vi "Camera Test Suite.vi"() -> ()   [LabVIEW 2015]
panel:
  out "Status":T1
  in  "Exposure":dbl=0.1
  in  "Save location":path
  out "Image":T2(plugin-control)
  in  "Test":bool
  in  "stop":bool
  in  "Function to test":T3(ring)
  in  "Camera vi path":path
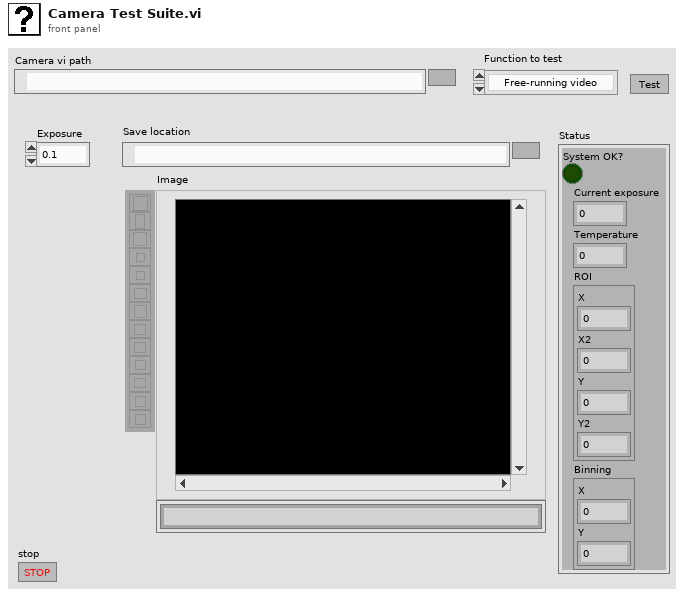
[diagram p1: front panel]
types:
  T1 = cluster{"System OK?":bool, "Current exposure":dbl, "Temperature":dbl, "ROI":cluster{"X":u32, "X2":u32, "Y":u32, "Y2":u32}, "Binning":cluster{"X":u32, "Y":u32}}
  T2 = typedef "IMAQ Image.ctl" = refnum<image>
  T3 = enum16{"Free-running video", "Capture 1 frame", "Capture 10 frames", "Settings", "Change exposure", "Get status"}
  T4 = typedef "Image Type" = u32
  T5 = enum16{"Initialize", "Shut down", "Set capture mode", "Set exposure", "Trigger and read", "Get status", "Other settings"}
  T6 = cluster{"New Image":T2, "Image":refnum<vi>, "FPS target":dbl}
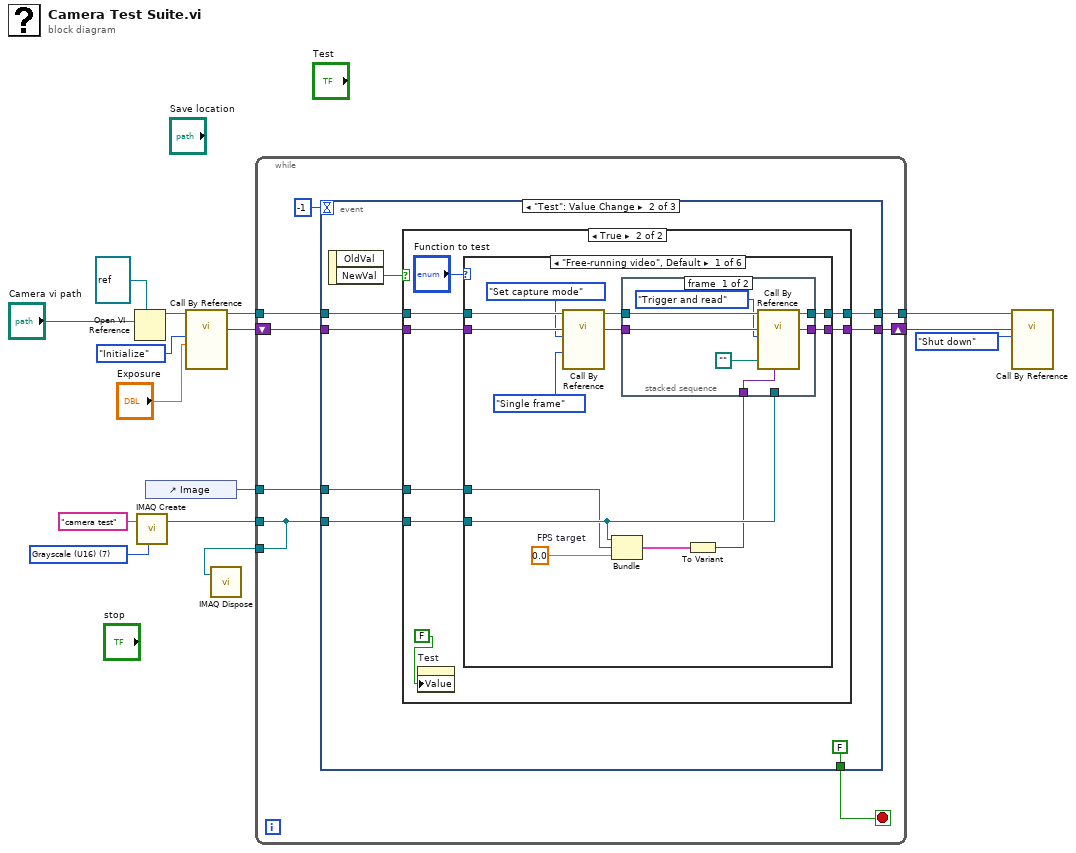
[diagram p0: block diagram]
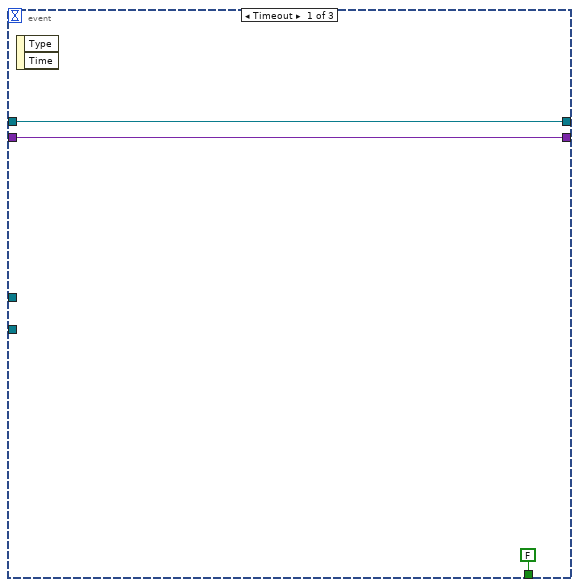
[diagram p2: hidden frame]
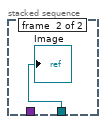
[diagram p4: hidden frame]
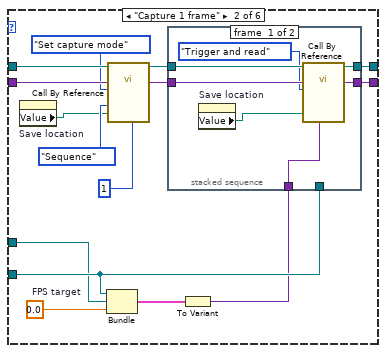
[diagram p5: hidden frame]
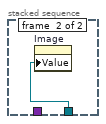
[diagram p6: hidden frame]
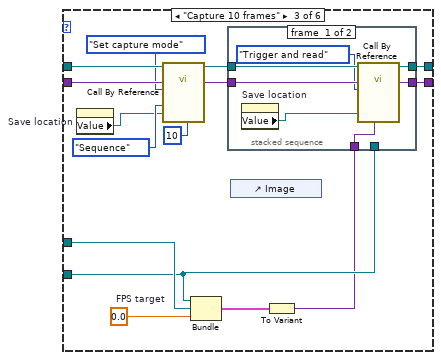
[diagram p7: hidden frame]
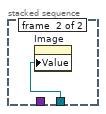
[diagram p8: hidden frame]
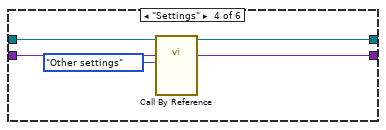
[diagram p9: hidden frame]
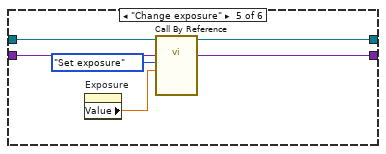
[diagram p10: hidden frame]
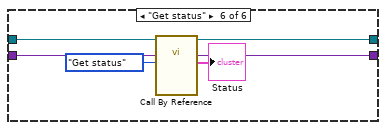
[diagram p11: hidden frame]
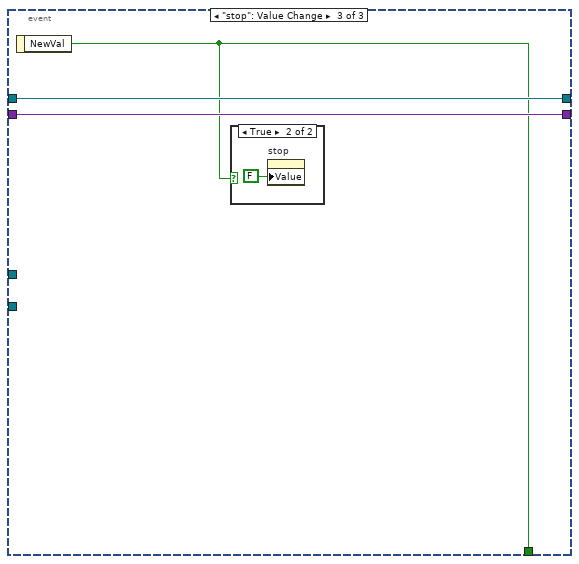
[diagram p12: hidden frame]
diagram:
  w5 = T4 7 items=["Grayscale (U8)", "Grayscale (I16)", "Grayscale (SGL)", "Complex (CSG)", "RGB (U32)", "HSL (U32)", "RGB (U64)", "Grayscale (U16)"] ("Image Type")
  n1 = Open VI Reference(type specifier VI Refnum (for type only)=refnum<vi> refnum, vi path="Camera vi path") -> (vi reference=w13:refnum<vi>)  [unwired: 4 in, 1 out]
  n2 = call "IMAQ Create"("Image Name"="camera test", "Image Type"=w5) -> ("New Image"=w4:T2)  [unwired: 3 in, 1 out]
  n3 = control-ref of="Image"() -> (w1:refnum<vi>)
  n4 = call-by-ref "?"(reference=w13, "Exposure time (s)"="Exposure", "Operation"=T5."Initialize") -> (reference out=w10:refnum<vi>, "Camera-specific out"=w8:variant)  [unwired: 9 in, 2 out]
  n5 = while {
    tunnel: w10 -> [w21]
    tunnel: [w22] -> w12
    shift-right: [w20] -> w7
    shift-left: w8 -> [w19]
    tunnel: w4 -> [w18]
    tunnel: [w18] -> w3
    tunnel: w1 -> [w16]
    stop <- w17 stop-if-true
    n6 = event shown="[1] \"Test\": Value Change" {
      selector: _ -> [_ _ _]
      dyn-events: _ -> [_ _ _]
      timeout: -1 -> [_ _ _]
      tunnel: [w26 w34 w131] -> w22
      tunnel: w21 -> [w26 w33 w131]
      tunnel: [w25 w32 w130] -> w20
      tunnel: w19 -> [w25 w31 w130]
      tunnel: w18 -> [_ w29 _]
      tunnel: [FALSE ("NewVal") FALSE ("NewVal") w129] -> w17
      tunnel: w16 -> [_ w27 _]
      event Timeout {
        n7 = event-data() -> ()  [unwired: 1 in, 2 out]
      }
      event "Test": Value Change {
        n8 = event-data() -> ("NewVal"=w30:bool)  [unwired: 1 in, 1 out]
        n9 = case shown="True" w30 {
          tunnel: [w36 w43] -> w34
          tunnel: w33 -> [w36 w42]
          tunnel: [w35 w41] -> w32
          tunnel: w31 -> [w35 w40]
          tunnel: w29 -> [_ w38]
          tunnel: w27 -> [_ w37]
          frame False {
          }
          frame True {
            n10 = property on="Test" class="Bool (strict)"("Value"=FALSE) -> ()  [unwired: 2 in, 2 out]
            n11 = case shown="\"Free-running video\", Default" "Function to test" {
              tunnel: [w52 w75 w98 w115 w121 w127] -> w43
              tunnel: w42 -> [w57 w80 w103 w116 w122 w128]
              tunnel: [w50 w73 w96 w113 w119 w125] -> w41
              tunnel: w40 -> [w56 w79 w102 w114 w120 w126]
              tunnel: w38 -> [w47 w70 w90 _ _ _]
              tunnel: w37 -> [w46 w69 w91 _ _ _]
              frame "Free-running video", Default {
                w49 = 0.0  # FPS target
                n12 = call-by-ref "?"(reference=w57, "Camera-specific in"=w56, "Capture mode"=enum16{"Single frame", "Sequence"}."Single frame", "Operation"=T5."Set capture mode") -> (reference out=w53:refnum<vi>, "Camera-specific out"=w51:variant)  [unwired: 8 in, 2 out]
                n13 = Bundle("New Image"=w47, "Image"=w46, "FPS target"=w49) -> (w48:T6)  [unwired: 1 in]
                n14 = To Variant(anything=w48) -> (Variant=w45:variant)
                n15 = stacked-sequence {
                  tunnel: w53 -> [w64 _]
                  tunnel: [w63 _] -> w52
                  tunnel: w51 -> [w62 _]
                  tunnel: [w61 _] -> w50
                  tunnel: w47 -> [_ w65]
                  tunnel: w45 -> [w58 _]
                  frame #0 {
                    n16 = call-by-ref "?"(reference=w64, "Image in"=w58, "Camera-specific in"=w62, "Save path"=path "", "Operation"=T5."Trigger and read") -> (reference out=w63:refnum<vi>, "Camera-specific out"=w61:variant)  [unwired: 7 in, 2 out]
                  }
                  frame #1 {
                    "Image" <- w65
                  }
                }
              }
              frame "Capture 1 frame" {
                w68 = 0.0  # FPS target
                n17 = property on="Save location" class="Path"() -> ("Value"=w71:path)  [unwired: 2 in, 2 out]
                n18 = Bundle("New Image"=w70, "Image"=w69, "FPS target"=w68) -> (w67:T6)  [unwired: 1 in]
                n19 = call-by-ref "?"(reference=w80, "Frames in sequence"=u32 1, "Camera-specific in"=w79, "Save path"=w71, "Capture mode"=enum16{"Single frame", "Sequence"}."Sequence", "Operation"=T5."Set capture mode") -> (reference out=w76:refnum<vi>, "Camera-specific out"=w74:variant)  [unwired: 6 in, 2 out]
                n20 = To Variant(anything=w67) -> (Variant=w66:variant)
                n21 = stacked-sequence {
                  tunnel: w76 -> [w87 _]
                  tunnel: [w86 _] -> w75
                  tunnel: w74 -> [w85 _]
                  tunnel: [w84 _] -> w73
                  tunnel: w70 -> [_ w88]
                  tunnel: w66 -> [w81 _]
                  frame #0 {
                    n22 = property on="Save location" class="Path"() -> ("Value"=w82:path)  [unwired: 2 in, 2 out]
                    n23 = call-by-ref "?"(reference=w87, "Image in"=w81, "Camera-specific in"=w85, "Save path"=w82, "Operation"=T5."Trigger and read") -> (reference out=w86:refnum<vi>, "Camera-specific out"=w84:variant)  [unwired: 7 in, 2 out]
                  }
                  frame #1 {
                    n24 = property on="Image" class="ImageControl"("Value"=w88) -> ()  [unwired: 2 in, 2 out]
                  }
                }
              }
              frame "Capture 10 frames" {
                w93 = 0.0  # FPS target
                n25 = property on="Save location" class="Path"() -> ("Value"=w94:path)  [unwired: 2 in, 2 out]
                n26 = call-by-ref "?"(reference=w103, "Frames in sequence"=u32 10, "Camera-specific in"=w102, "Save path"=w94, "Capture mode"=enum16{"Single frame", "Sequence"}."Sequence", "Operation"=T5."Set capture mode") -> (reference out=w99:refnum<vi>, "Camera-specific out"=w97:variant)  [unwired: 6 in, 2 out]
                n27 = Bundle("New Image"=w90, "Image"=w91, "FPS target"=w93) -> (w92:T6)  [unwired: 1 in]
                n28 = control-ref of="Image"() -> ()  [unwired: 1 out]
                n29 = To Variant(anything=w92) -> (Variant=w89:variant)
                n30 = stacked-sequence {
                  tunnel: w99 -> [w110 _]
                  tunnel: [w109 _] -> w98
                  tunnel: w97 -> [w108 _]
                  tunnel: [w107 _] -> w96
                  tunnel: w90 -> [_ w111]
                  tunnel: w89 -> [w104 _]
                  frame #0 {
                    n31 = property on="Save location" class="Path"() -> ("Value"=w105:path)  [unwired: 2 in, 2 out]
                    n32 = call-by-ref "?"(reference=w110, "Image in"=w104, "Camera-specific in"=w108, "Save path"=w105, "Operation"=T5."Trigger and read") -> (reference out=w109:refnum<vi>, "Camera-specific out"=w107:variant)  [unwired: 7 in, 2 out]
                  }
                  frame #1 {
                    n33 = property on="Image" class="ImageControl"("Value"=w111) -> ()  [unwired: 2 in, 2 out]
                  }
                }
              }
              frame "Settings" {
                n34 = call-by-ref "?"(reference=w116, "Camera-specific in"=w114, "Operation"=T5."Other settings") -> (reference out=w115:refnum<vi>, "Camera-specific out"=w113:variant)  [unwired: 9 in, 2 out]
              }
              frame "Change exposure" {
                n35 = property on="Exposure" class="DigNum (strict)"() -> ("Value"=w117:dbl)  [unwired: 2 in, 2 out]
                n36 = call-by-ref "?"(reference=w122, "Camera-specific in"=w120, "Exposure time (s)"=w117, "Operation"=T5."Set exposure") -> (reference out=w121:refnum<vi>, "Camera-specific out"=w119:variant)  [unwired: 8 in, 2 out]
              }
              frame "Get status" {
                n37 = call-by-ref "?"(reference=w128, "Camera-specific in"=w126, "Operation"=T5."Get status") -> (reference out=w127:refnum<vi>, "Status"=→"Status":T1, "Camera-specific out"=w125:variant)  [unwired: 9 in, 1 out]
              }
            }
          }
        }
      }
      event "stop": Value Change {
        n38 = event-data() -> ("NewVal"=w129:bool)  [unwired: 1 in]
        n39 = case shown="True" w129 {
          frame False {
          }
          frame True {
            n40 = property on="stop" class="Bool (strict)"("Value"=FALSE ("stop")) -> ()  [unwired: 2 in, 2 out]
          }
        }
      }
    }
  }
  n41 = call "IMAQ Dispose"("Image"=w3) -> ()  [unwired: 5 in, 1 out]
  n42 = call-by-ref "?"(reference=w12, "Camera-specific in"=w7, "Operation"=T5."Shut down") -> ()  [unwired: 9 in, 4 out]
